vi "Destroy.vi"(8 "error in (no error)":errorcluster, 11 "CIFTag in":refnum<class "CIF_NIChn.lvclass">) -> (0 "error out":errorcluster, 3 "CIFTag out":refnum<class "CIF_NIChn.lvclass">)   [LabVIEW 2021, in "CIF_NIChn.lvclass"]
uses:
  CIF_NIChn.lvclass
  CIF_NIChn.lvclass/CIF_NIChn.ctl
  <vilib>/CIFChannels/SubVIs/CIFServices Fill In Error Info Ex.vi
  <vilib>/CIFChannels/SubVIs/Get dll Path.vi
  <vilib>/CIFChannels/SubVIs/Append Error Location.vi
  <vilib>/CIFChannels/CIFChannelCore.lvlib
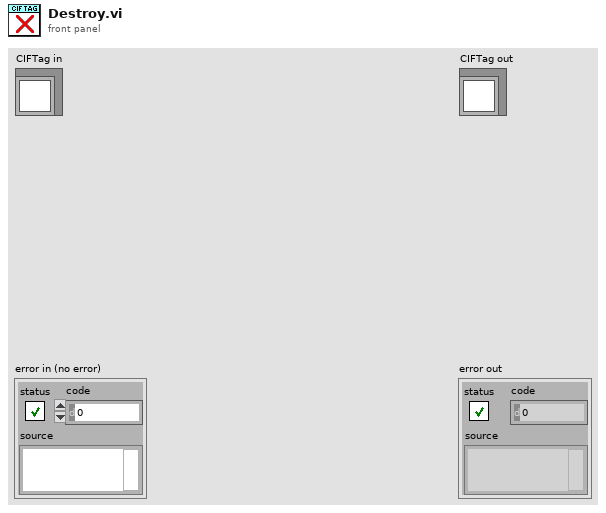
[diagram p1: front panel]
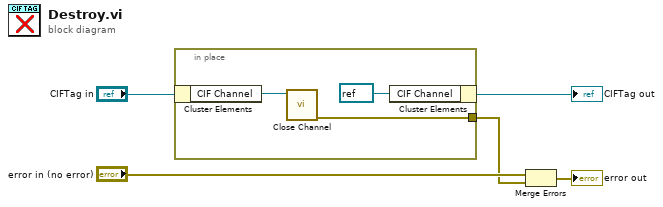
[diagram p0: block diagram]
diagram:
  n1 = in-place {
    in-place-border: [w6] -> w2
    n2 = in-place-cluster #1("CIFTag in") -> ("CIF Channel"=w8:refnum<k21>)
    n3 = call <vilib>:"Close Channel.vi"("CIF Channel"=w8) -> ("error out"=w6:errorcluster)  [unwired: 10 in]
    n4 = in-place-cluster #1("CIF Channel"=refnum<k21> refnum) -> (→"CIFTag out":refnum<class "CIF_NIChn.lvclass">)
  }
  n5 = Merge Errors("error in (no error)", w2) -> (→"error out":errorcluster)
